vi "Read SV_Publisher.vi"(11 "Stand in":refnum<class "Stand.lvclass">) -> (2 "SV_Publisher.lvclass":refnum<class "SV_Publisher.lvclass">)   [LabVIEW 2019, in "Stand.lvclass"]
uses:
  Stand.lvclass
  SV_Puplisher_class/SV_Publisher.lvclass
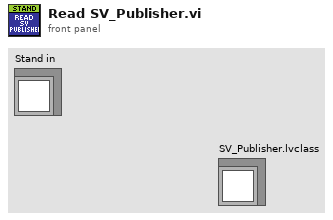
[diagram p1: front panel]
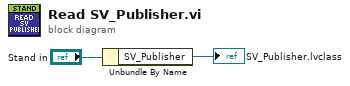
[diagram p0: block diagram]
diagram:
  n1 = Unbundle By Name("Stand in") -> ("SV_Publisher"=→"SV_Publisher.lvclass":refnum<class "SV_Publisher.lvclass">)
